vi "FGV EX 2 USE CASE.vi"() -> ()   [LabVIEW 2022 SP3]
panel:
  out "Waveform Chart 2":dbl(graph)
  out "Waveform Chart":dbl(graph)
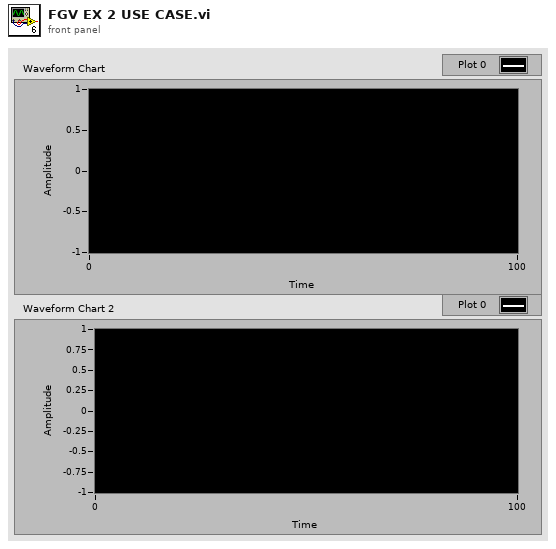
[diagram p1: front panel]
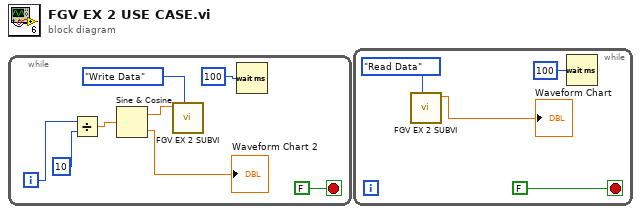
[diagram p0: block diagram]
diagram:
  n1 = while {
    i -> [w8]
    stop <- FALSE stop-if-true
    n2 = Divide(x=w8, y=10) -> (x/y=w6:dbl)
    n3 = Sine & Cosine(0:w6) -> (1:w5:dbl, 2:→"Waveform Chart 2":dbl)
    n4 = call "FGV EX 2 SUBVI.vi"("Enum"=enum16{"Write Data", "Read Data"}."Write Data", "input in"=w5) -> ()  [unwired: 9 in, 1 out]
    n5 = Wait (ms)(milliseconds to wait=u32 100) -> ()  [unwired: 1 out]
  }
  n6 = while {
    stop <- FALSE stop-if-true
    n7 = call "FGV EX 2 SUBVI.vi"("Enum"=enum16{"Write Data", "Read Data"}."Read Data") -> ("input out"=→"Waveform Chart":dbl)  [unwired: 10 in]
    n8 = Wait (ms)(milliseconds to wait=u32 100) -> ()  [unwired: 1 out]
  }
